vi "sub_dt.vi"() -> (3 "dt":u32)   [LabVIEW 2013]
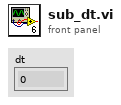
[diagram p1: front panel]
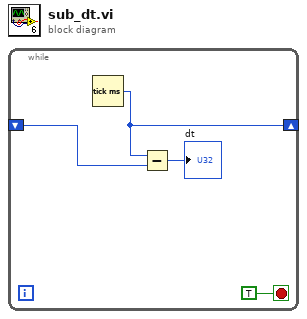
[diagram p0: block diagram]
diagram:
  n1 = while {
    shift-right: [w3] -> _
    shift-left: _ -> [w2]
    stop <- TRUE stop-if-true
    n2 = Tick Count (ms)() -> (millisecond timer value=w3:u32)
    n3 = Subtract(x=w3, y=w2) -> (x-y=→"dt":u32)
  }
